vi "Material-Subtract-ToApply.vi"(0 "Material-RunTest in":refnum<class "Material-RunTest.lvclass">, 1 "Description":string) -> (5 "Part Number not Valid for sheet":bool, 6 "Material-RunTest out":refnum<class "Material-RunTest.lvclass">)   [LabVIEW 2013, in "Material-RunTest.lvclass"]
uses:
  Material-RunTest.lvclass
  Material-RunTest.lvclass/Material-RunTest.ctl
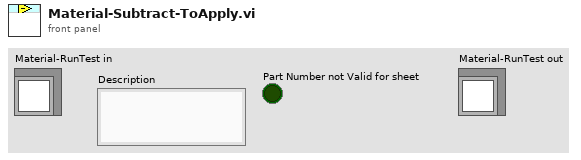
[diagram p1: front panel]
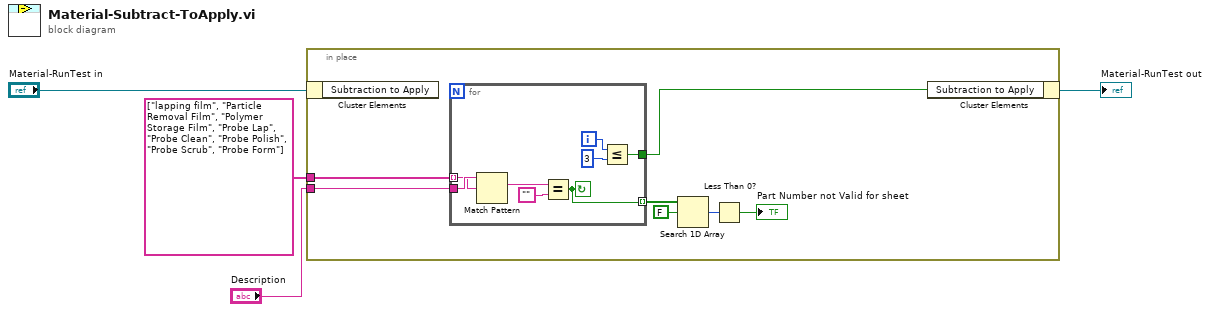
[diagram p0: block diagram]
diagram:
  n1 = in-place {
    in-place-border: string[] ["lapping film", "Particle Removal Film", "Polymer Storage Film", "Probe Lap", "Probe Clean", "Probe Polish", "Probe Scrub", "Probe Form"] -> [w11]
    in-place-border: "Description" -> [w10]
    n2 = in-place-cluster #1("Material-RunTest in") -> ()  [unwired: 1 out]
    n3 = for {
      tunnel: w11 -> [w12] mode=indexing
      tunnel: w10 -> [w13]
      tunnel: [w15] -> w9
      tunnel: [w14] -> w8 mode=indexing
      i -> [w19]
      stop <- w14 continue-if-true
      n4 = Match Pattern(string=w13, regular expression=w12) -> (match substring=w17:string)  [unwired: 1 in, 3 out]
      n5 = Equal?(x=w17, y="") -> (x = y?=w14:bool)
      n6 = Less Or Equal?(x=w19, y=3 ("x")) -> (x <= y?=w15:bool)
    }
    n7 = Search 1D Array(1D array=w8, element=FALSE) -> (index of element=w6:i32)  [unwired: 1 in]
    n8 = Less Than 0?(x=w6) -> (x < 0?=→"Part Number not Valid for sheet":bool)
    n9 = in-place-cluster #1("Subtraction to Apply"=w9) -> (→"Material-RunTest out":refnum<class "Material-RunTest.lvclass">)
  }
